vi "Test XY Scanning with Alazar.vi"() -> ()   [LabVIEW 2018]
uses:
  Hardware Mfg/AlazarTech SDK/Controls/Alazar Engine Actions.ctl
  <vilib>/ErrorRing/Error Ring.xnode
  General/Controls/Queue Manager Actions.ctl
  General/data manager action.ctl
  General/Controls/Optical Parameters.ctl
  General/Controls/Vibratome Parameters.ctl
  General/Controls/Translation Stage Types.ctl
  Hardware Mfg/Thorlabs Translation Stages/Controls/Translation Stage Cluster.ctl
  General/Controls/Translation Stage Parameters.ctl
  General/Controls/Scan Direction.ctl
  General/Controls/Imaging Parameters.ctl
  General/Controls/System Parameters.ctl
  Hardware Mfg/AlazarTech SDK/Controls/Clock Controls.ctl
  Hardware Mfg/AlazarTech SDK/Controls/Alazar Device ID.ctl
  Hardware Mfg/AlazarTech SDK/Controls/Channel Input Controls.ctl
  Hardware Mfg/AlazarTech SDK/Controls/Trigger Engine Controls.ctl
  Hardware Mfg/AlazarTech SDK/Controls/General Trigger Settings.ctl
  Hardware Mfg/AlazarTech SDK/Controls/Alazar Acquisition Settings.ctl
  General/type defines/file type.ctl
  General/Controls/Control cluster.ctl
panel:
  out "# save":i32
  out "# display":i32
  in  "save?":bool
  out "Image":T1(plugin-control)
  in  "Cluster":T2={"FFT value magnification"=1000.0, "max queue size (-1, unlimited)"=-1, "File Type"=enum."Tiff", "file path"=path "C:/Users/BoasLab/Documents/Data/Alazar data/B-line/data/test.tif", "#A-lines to save"=2048, "#Z pixels to save"=2048, "ImageDescription"="", "Convert to U16?"=FALSE} {"FFT value magnification" min=0.0 max=10000.0 step=0.001 format="%.4f"}
  out "error out":errorcluster
  in  "Acq Settings":T4={"Window Type"=1, "Record Length"=1440, "Footer"=0, "Output Format"=11, "Offset"=0, "Records Per Buffer"=2048, "Samples per record"=2048, "Records Count (Records/Acq)"=2147483647} {"Window Type" items=["DSP_WINDOW_NONE", "DSP_WINDOW_HANNING", "DSP_WINDOW_HAMMING", "DSP_WINDOW_BLACKMAN", "DSP_WINDOW_BLACKMAN_HARRIS", "DSP_WINDOW_BARTLETT"]; "Footer" items=["FOOTER_NONE", "FOOTER_NPT"]; "Output Format" items=["FLOAT_AMP2"=10, "FLOAT_LOG"=11]}
  in  "Trigger Settings":T7={"General Trigger Settings"={"Trigger Operation"=0, "Coupling ID"=2, "Range ID"=2, "Delay"=0, "Timeout Ticks"=0, "Mode"=1, "Parameter"=1}, "Trigger Engine 1"={"Trigger Engine"=0, "Source"=2, "Slope"=1, "Level"=140}, "Trigger Engine 2"={"Trigger Engine"=1, "Source"=3, "Slope"=1, "Level"=140}} {"General Trigger Settings"."Trigger Operation" items=["J", "K", "J OR K", "J AND K", "J XOR K", "J AND NOT K", "NOT J AND K"]; "General Trigger Settings"."Coupling ID" items=["AC"=1, "DC"=2]; "General Trigger Settings"."Range ID" items=["5 V", "1 V", "TTL"]; "Trigger Engine 1"."Trigger Engine" items=["J", "K"]; "Trigger Engine 1"."Source" items=["A", "B", "External", "Disable", "C", "D"]; "Trigger Engine 1"."Slope" items=["Positive"=1, "Negative"=2]; "Trigger Engine 2"."Trigger Engine" items=["J", "K"]; "Trigger Engine 2"."Source" items=["A", "B", "External", "Disable", "C", "D"]; "Trigger Engine 2"."Slope" items=["Positive"=1, "Negative"=2]}
  in  "Ch B Input Control":T8={"Channel"=2, "Coupling"=2, "Range"=10, "Impedance"=2} {"Channel" items=["A"=1, "B"=2, "C"=4, "D"=8]; "Coupling" items=["AC"=1, "DC"=2]; "Range" items=["20 mV"=1, "40 mV"=2, "50 mV"=3, "80 mV"=4, "100 mV"=5, "200 mV"=6, "400 mV"=7, "500 mV"=8, "800 mV"=9, "1 V"=10, "1.25 V"=33, "2 V"=11, "4 V"=12, "5 V"=13, "8 V"=14, "10 V"=15, "20 V"=16]; "Impedance" items=["1 MOhm"=1, "50 Ohm"=2, ""=0]}
  in  "Ch A Input Control":T8={"Channel"=1, "Coupling"=2, "Range"=10, "Impedance"=2} {"Channel" items=["A"=1, "B"=2, "C"=4, "D"=8]; "Coupling" items=["AC"=1, "DC"=2]; "Range" items=["20 mV"=1, "40 mV"=2, "50 mV"=3, "80 mV"=4, "100 mV"=5, "200 mV"=6, "400 mV"=7, "500 mV"=8, "800 mV"=9, "1 V"=10, "1.25 V"=33, "2 V"=11, "4 V"=12, "5 V"=13, "8 V"=14, "10 V"=15, "20 V"=16]; "Impedance" items=["1 MOhm"=1, "50 Ohm"=2, ""=0]}
  in  "Device ID":T9={"System ID"=1, "Board ID"=1}
  in  "Capture Clock":T10={"Sample Rate"=100, "Decimation"=0, "Source"=2, "Edge"=0} {"Edge" items=["Rising", "Falling"]; "Source" items=["Internal"=1, "Fast External"=2, "Medium External"=3, "Slow External"=4, "External AC"=5, "External DC"=6, "External 10MHz"=7]}
  out "Acquisition":i32
  in  "stop":bool
  in  "System Parameters":T11={"Optical Parameters"={"Obj. Focal Length [mm]"=45.0, "Scan Lens EFL[mm]"=59.5, "Tube Lens EFL[mm]"=205.0, "Galvo V Range (+/-)"=10.0, "Galvo Max Half Angle [Deg]"=19.0, "Max Galvo Range[%]"=0.0}, "Vibratome"={"Z Bottom [mm]"=0.0, "Pre Cut Dwell [s]"=0.0, "Blade Frequency [RPM]"=0, "Slice Speed [mm/s]"=0.0, "Post Cut Dwell [s]"=0.0, "Ramp Time [s]"=0.0, "Start X [mm]"=0.0, "Start Y [mm]"=0.0, "Slice Length [mm]"=0.0, "Slice Axis"=enum."Y Axis", "Controller VISA Ref"="COM4"}, "Table Stages"={"X Stage"={"Position"=0.0, "Is.Enabled?"=FALSE, "Is.Connected?"=FALSE, "Device SN"="45876539", "AccelerationMaximum"=0.0, "VelocityMaximum"=0.0, "Acceleration"=0.0, "Velocity"=0.0, "waitTimeout (ms)"=0, "Model"=enum."None", "Is.Homed?"=FALSE}, "Y Stage"={"Position"=0.0, "Is.Enabled?"=FALSE, "Is.Connected?"=FALSE, "Device SN"="45876539", "AccelerationMaximum"=0.0, "VelocityMaximum"=0.0, "Acceleration"=0.0, "Velocity"=0.0, "waitTimeout (ms)"=0, "Model"=enum."None", "Is.Homed?"=FALSE}, "Z Stage"={"Position"=0.0, "Is.Enabled?"=FALSE, "Is.Connected?"=FALSE, "Device SN"="45876539", "AccelerationMaximum"=0.0, "VelocityMaximum"=0.0, "Acceleration"=0.0, "Velocity"=0.0, "waitTimeout (ms)"=0, "Model"=enum."None", "Is.Homed?"=FALSE}}, "Imaging Parameter"={"Raster Scan Direction"=enum."Uni Directional", "Pixel Dwell Time [Clock Cycles]"=1, "Flyback Time [Clock Cycles]"=200, "XY Center [um]"={"X"=1.0, "Y"=1.0}, "Pixel Step Size [um]"=2.5, "XY Image Size"=enum."2048 x 2048", "Custom"=FALSE, "Custom Size"={"X"=10, "Y"=10}, "Line Averages"=1}} {"Imaging Parameter"."Line Averages" min=1 max=30 step=1; "Imaging Parameter"."Flyback Time [Clock Cycles]" max=1000 step=1; "Imaging Parameter"."Pixel Step Size [um]" min=0.0 max=10.0 step=0.01; "Imaging Parameter"."Custom Size"."Y" min=1 max=30 step=1; "Imaging Parameter"."Custom Size"."X" min=1 max=30 step=1; "Imaging Parameter"."XY Center [um]"."Y" min=1.0 max=30.0 step=1.0; "Imaging Parameter"."XY Center [um]"."X" min=1.0 max=30.0 step=1.0; "Imaging Parameter"."Pixel Dwell Time [Clock Cycles]" max=10 step=1}
  in  "Galvo HW Parameters":T19={"Analog Out Channel"="GalvoCtrl/ao0,GalvoCtrl/ao1", "Min Voltage"=-10.0, "Max Voltage"=10.0, "Pixel Clock Source"="/GalvoCtrl/PFI0", "Sample Rate"=1000.0, "Line Clock Out Ch"="GalvoCtrl/port0/line0"}
  # "X"
  # "X"
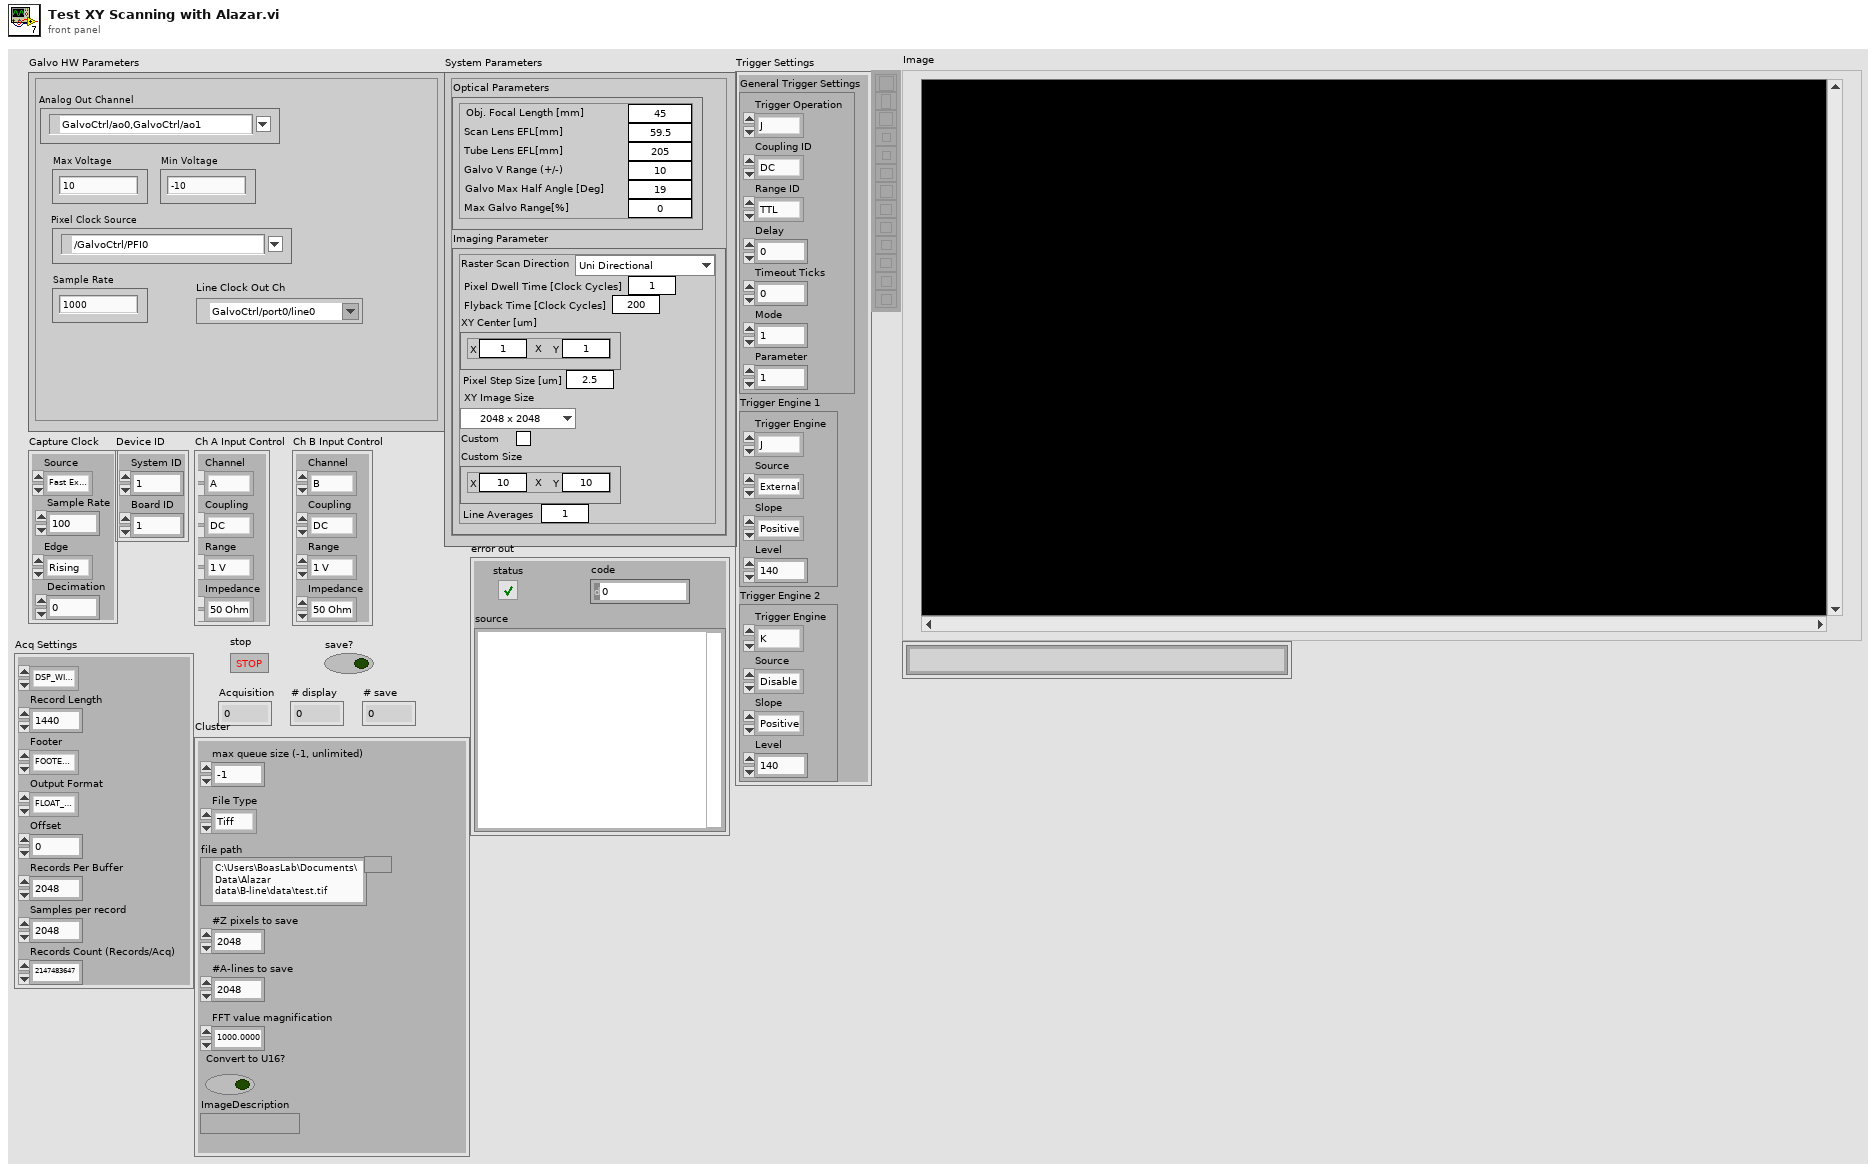
[diagram p1: front panel]
types:
  T1 = typedef "IMAQ Image.ctl" = refnum<image>
  T2 = typedef "Control cluster.ctl" = cluster{"FFT value magnification":dbl, "max queue size (-1, unlimited)":i32, "File Type":T3, "file path":path, "#A-lines to save":u32, "#Z pixels to save":u32, "ImageDescription":string, "Convert to U16?":bool}
  T3 = typedef "file type.ctl" = enum16{"text", "Tiff", "binary"}
  T4 = typedef "Alazar Acquisition Settings.ctl" = cluster{"Window Type":u32, "Record Length":u32, "Footer":u32, "Output Format":u32, "Offset":u32, "Records Per Buffer":u32, "Samples per record":u32, "Records Count (Records/Acq)":u32}
  T5 = typedef "General Trigger Settings.ctl" = cluster{"Trigger Operation":u32, "Coupling ID":u32, "Range ID":u32, "Delay":u32, "Timeout Ticks":u32, "Mode":u32, "Parameter":u32}
  T6 = typedef "Trigger Engine Controls.ctl" = cluster{"Trigger Engine":u32, "Source":u32, "Slope":u32, "Level":u32}
  T7 = cluster{"General Trigger Settings":T5, "Trigger Engine 1":T6, "Trigger Engine 2":T6}
  T8 = typedef "Channel Input Controls.ctl" = cluster{"Channel":u8, "Coupling":u32, "Range":u32, "Impedance":u32}
  T9 = typedef "Alazar Device ID.ctl" = cluster{"System ID":u32, "Board ID":u32}
  T10 = typedef "Clock Controls.ctl" = cluster{"Sample Rate":u32, "Decimation":u32, "Source":u32, "Edge":u32}
  T11 = typedef "System Parameters.ctl" = cluster{"Optical Parameters":T12, "Vibratome":T13, "Table Stages":T14, "Imaging Parameter":T17}
  T12 = typedef "Optical Parameters.ctl" = cluster{"Obj. Focal Length [mm]":dbl, "Scan Lens EFL[mm]":dbl, "Tube Lens EFL[mm]":dbl, "Galvo V Range (+/-)":dbl, "Galvo Max Half Angle [Deg]":dbl, "Max Galvo Range[%]":dbl}
  T13 = typedef "Vibratome Parameters.ctl" = cluster{"Z Bottom [mm]":dbl, "Pre Cut Dwell [s]":dbl, "Blade Frequency [RPM]":u16, "Slice Speed [mm/s]":dbl, "Post Cut Dwell [s]":dbl, "Ramp Time [s]":dbl, "Start X [mm]":dbl, "Start Y [mm]":dbl, "Slice Length [mm]":dbl, "Slice Axis":enum16{"X Axis", "Y Axis", "Z Axis"}, "Controller VISA Ref":refnum<visa-resource-name>}
  T14 = typedef "Translation Stage Parameters.ctl" = cluster{"X Stage":T15, "Y Stage":T15, "Z Stage":T15}
  T15 = typedef "Translation Stage Cluster.ctl" = cluster{"Position":dbl, "Is.Enabled?":bool, "Is.Connected?":bool, "Device SN":string, "AccelerationMaximum":dbl, "VelocityMaximum":dbl, "Acceleration":dbl, "Velocity":dbl, "waitTimeout (ms)":i32, "Model":T16, "Is.Homed?":bool}
  T16 = typedef "Translation Stage Types.ctl" = enum16{"None", "Thorlabs LTS", "Thorlabs MLJ"}
  T17 = typedef "Imaging Parameters.ctl" = cluster{"Raster Scan Direction":T18, "Pixel Dwell Time [Clock Cycles]":u16, "Flyback Time [Clock Cycles]":u16, "XY Center [um]":cluster{"X":dbl, "Y":dbl}, "Pixel Step Size [um]":dbl, "XY Image Size":enum16{"32 x 32", "64 x 64", "128 x 128", "256 x 256", "512 x 512", "1024 x 1024", "2048 x 2048"}, "Custom":bool, "Custom Size":cluster{"X":u16, "Y":u16}, "Line Averages":u8}
  T18 = typedef "Scan Direction.ctl" = enum16{"Uni Directional", "Bi Directional", "None"}
  T19 = cluster{"Analog Out Channel":tag, "Min Voltage":dbl, "Max Voltage":dbl, "Pixel Clock Source":tag, "Sample Rate":dbl, "Line Clock Out Ch":tag}
  T20 = typedef "Queue Manager Actions.ctl" = enum16{"Init", "Enqueue", "Enqueue All", "Preview Queue", "Dequeue", "Get Status", "Flush Queue", "Flush All Queues", "Release All Queues", "Release Queue", "Enqueue at Opposite End"}
  T21 = typedef "Alazar Engine Actions.ctl" = enum16{"Init", "Config Clock", "Config Ch", "Config Trig", "Config Non-FFT Acq.", "Non-FFT Acquire", "Load background from Non-FFT buffer", "enable background subtrac", "disable background subtrac", "load background from file", "load background from elsewhere", "start acquire", "background subtraction", "Config Acq.", "Acquire", "UnInit"}
  T22 = enum16{"Init", "Calc & Write Scan Pattern", "Start Galvo Task", "Is Task Done?", "Stop Galvo", "Uninit"}
  T23 = typedef "data manager action.ctl" = enum16{"Init: open file", "save", "save as text", "Uninit: close file"}
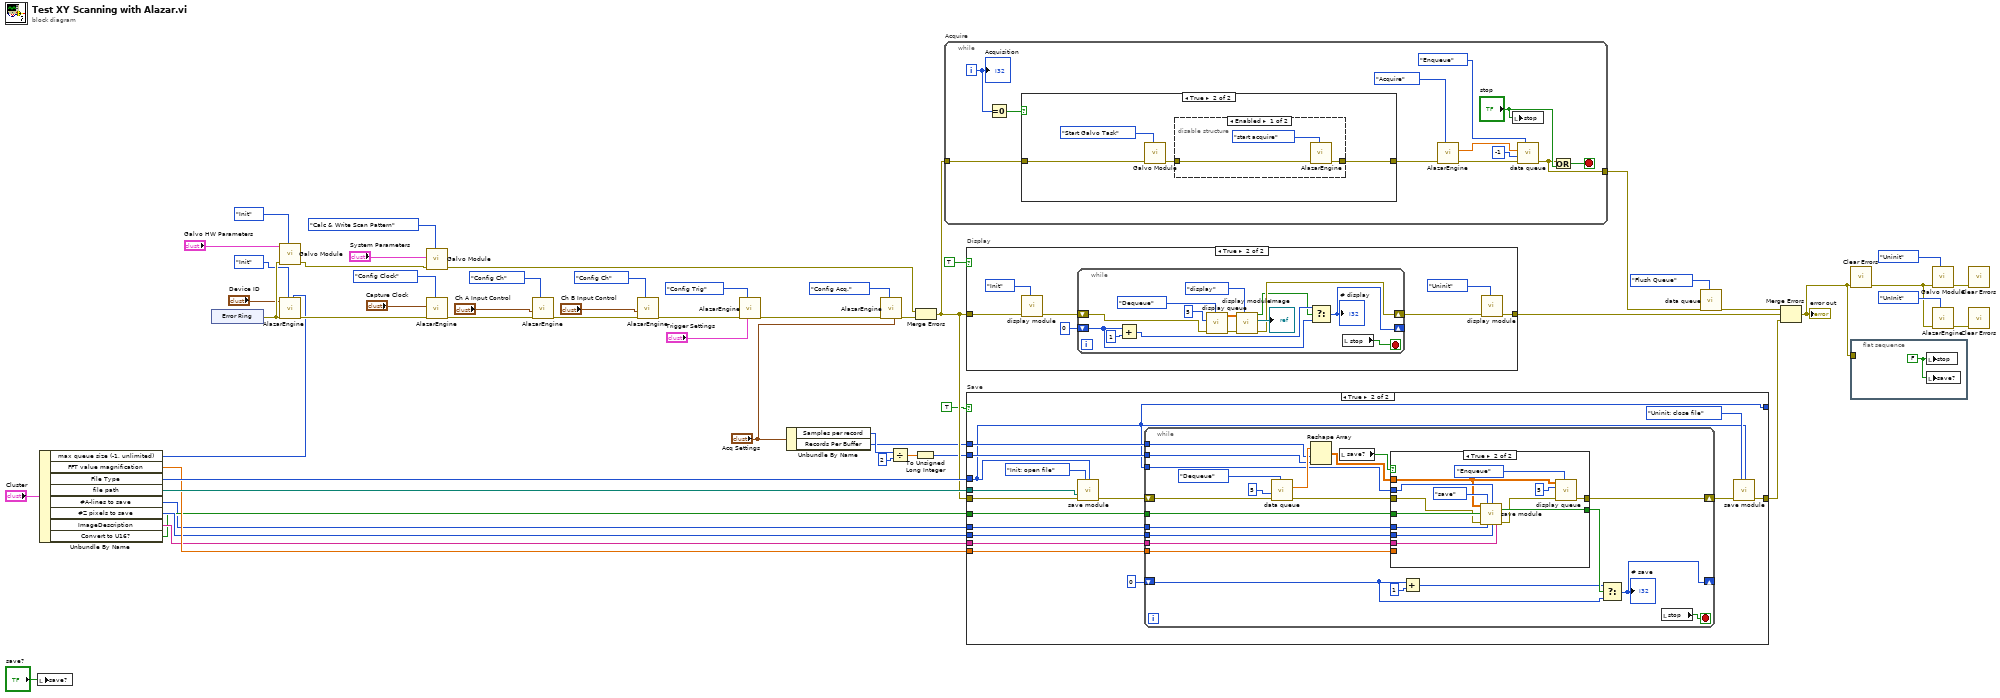
[diagram p0: block diagram]
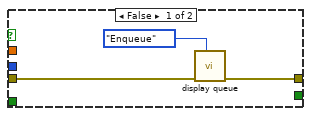
[diagram p3: hidden frame]
diagram:
  n1 = local write "save?"("save?") -> ()
  n2 = Unbundle By Name("Cluster") -> ("max queue size (-1, unlimited)"=w11:i32, "FFT value magnification"=w12:dbl, "File Type"=w16:T3, "file path"=w15:path, "#A-lines to save"=w3:u32, "#Z pixels to save"=w6:u32, "ImageDescription"=w5:string, "Convert to U16?"=w4:bool)
  n3 = xnode "Error Ring"() -> ("error out"=w45:errorcluster)
  n4 = call "Galvo Module.vi"("Action"=T22."Init", "error in (no error)"=w45, "Galvo HW Parameters"="Galvo HW Parameters") -> ("error out"=w52:errorcluster)  [unwired: 7 in, 1 out]
  n5 = call "AlazarEngine.vi"("max queue size (-1, unlimited)"=w11, "Action"=Alazar_Engine_Actions."Init", "error in (no error)"=w45, "Device ID"="Device ID") -> ("error out"=w48:errorcluster)  [unwired: 5 in, 2 out]
  n6 = call "Galvo Module.vi"("Action"=T22."Calc & Write Scan Pattern", "error in (no error)"=w52, "System Parameters"="System Parameters") -> ("error out"=w51:errorcluster)  [unwired: 7 in, 1 out]
  n7 = call "AlazarEngine.vi"("Action"=Alazar_Engine_Actions."Config Clock", "error in (no error)"=w48, "Capture Clock"="Capture Clock") -> ("error out"=w47:errorcluster)  [unwired: 6 in, 2 out]
  n8 = call "AlazarEngine.vi"("Action"=Alazar_Engine_Actions."Config Ch", "error in (no error)"=w47, "Ch Input Control"="Ch A Input Control") -> ("error out"=w46:errorcluster)  [unwired: 6 in, 2 out]
  n9 = call "AlazarEngine.vi"("Action"=Alazar_Engine_Actions."Config Ch", "error in (no error)"=w46, "Ch Input Control"="Ch B Input Control") -> ("error out"=w36:errorcluster)  [unwired: 6 in, 2 out]
  n10 = call "AlazarEngine.vi"("Trigger Settings"="Trigger Settings", "Action"=Alazar_Engine_Actions."Config Trig", "error in (no error)"=w36) -> ("error out"=w23:errorcluster)  [unwired: 6 in, 2 out]
  n11 = Unbundle By Name("Acq Settings") -> ("Samples per record"=w20:u32, "Records Per Buffer"=w1:u32)
  n12 = call "AlazarEngine.vi"("Acq Settings"="Acq Settings", "Action"=Alazar_Engine_Actions."Config Acq.", "error in (no error)"=w23) -> ("error out"=w32:errorcluster)  [unwired: 6 in, 2 out]
  n13 = Divide(x=w20, y=u32 2) -> (x/y=w18:dbl)
  n14 = To Unsigned Long Integer(number=w18) -> (unsigned 32bit integer=w2:u32)
  n15 = Merge Errors(w51, w32) -> (w10:errorcluster)
  n16 = while "Acquire" {
    tunnel: [w58] -> w24
    tunnel: w10 -> [w60]
    i -> [w59]
    stop <- w62 stop-if-true
    n17 = Equal To 0?(x=w59) -> (x = 0?=w66:bool)
    n18 = case shown="True" w66 {
      tunnel: [w67 w69] -> w65
      tunnel: w60 -> [w67 w68]
      frame False {
      }
      frame True {
        n19 = call "Galvo Module.vi"("Action"=T22."Start Galvo Task", "error in (no error)"=w68) -> ("error out"=w70:errorcluster)  [unwired: 8 in, 1 out]
        n20 = disable-structure shown="Enabled" {
          disable-tunnel: w70 -> [w74 w75]
          disable-tunnel: [w73 w75] -> w69
          frame Enabled {
            n21 = call "AlazarEngine.vi"("Action"=Alazar_Engine_Actions."start acquire", "error in (no error)"=w74) -> ("error out"=w73:errorcluster)  [unwired: 7 in, 2 out]
          }
          frame Disabled {
          }
        }
      }
    }
    n22 = call "AlazarEngine.vi"("Action"=Alazar_Engine_Actions."Acquire", "error in (no error)"=w65) -> ("error out"=w63:errorcluster, "Buffer"=w57:sgl[])  [unwired: 7 in, 1 out]
    n23 = local write "stop"("stop") -> ()
    n24 = call "data queue.vi"("Action"=Queue_Manager_Actions."Enqueue", "error in (no error)"=w63, "timeout in ms (-1)"=-1, "data in"=w57) -> ("error out"=w58:errorcluster)  [unwired: 4 in, 3 out]
    n25 = Or(x=w58, y="stop") -> (x .or. y?=w62:bool)
    "Acquisition" <- w59
  }
  n26 = case "Display" shown="True" TRUE {
    tunnel: [w76 w79] -> w14
    tunnel: w10 -> [w76 w78]
    frame False {
    }
    frame True {
      n27 = call "display module.vi"("Action"=enum16{"Init", "display", "Uninit"}."Init", "error in"=w78) -> ("error out"=w82:errorcluster)  [unwired: 7 in, 2 out]
      n28 = while {
        shift-right: [w94] -> w80
        shift-left: w82 -> [w88]
        shift-right: [w89] -> _
        shift-left: 0 -> [w90]
        stop <- w97 stop-if-true
        n29 = Add(x=w90, y=1) -> (x+y=w92:i32)
        n30 = call "display queue.vi"("Action"=Queue_Manager_Actions."Dequeue", "error in (no error)"=w88, "time out"=5 ("timeout in ms (-1)")) -> ("error out"=w85:errorcluster, "data out"=w84:sgl[][])  [unwired: 4 in, 3 out]
        n31 = call "display module.vi"("Action"=enum16{"Init", "display", "Uninit"}."display", "error in"=w85, "data in"=w84) -> ("error out"=w94:errorcluster, "Image"=→"Image":T1, "display successful?"=w91:bool)  [unwired: 6 in]
        n32 = Select(t=w92, s=w91, f=w90) -> (s? t:f=w89:i32)
        "# display" <- w89
        n33 = local read "stop"() -> (w97:bool)
      }
      n34 = call "display module.vi"("Action"=enum16{"Init", "display", "Uninit"}."Uninit", "error in"=w80) -> ("error out"=w79:errorcluster)  [unwired: 7 in, 2 out]
    }
  }
  n35 = case "Save" shown="True" TRUE {
    tunnel: w16 -> [_ w99]
    tunnel: w15 -> [_ w114]
    tunnel: [w98 w113] -> w13
    tunnel: w12 -> [_ w112]
    tunnel: w10 -> [w98 w111]
    tunnel: w6 -> [_ w107]
    tunnel: w5 -> [_ w104]
    tunnel: w4 -> [_ w105]
    tunnel: w3 -> [_ w106]
    tunnel: w2 -> [_ w103]
    tunnel: w1 -> [_ w102]
    tunnel: [_ w99] -> _
    frame False {
    }
    frame True {
      n36 = call "save module.vi"("action"=data_manager_action."Init: open file", "File Type"=w99, "file path and name"=w114, "error in (no error)"=w111) -> ("error out"=w110:errorcluster)  [unwired: 10 in, 1 out]
      n37 = while {
        tunnel: w112 -> [w135]
        shift-right: [w134] -> w109
        shift-left: w110 -> [w126]
        shift-right: [w129] -> _
        shift-left: 0 -> [w130]
        tunnel: w107 -> [w123]
        tunnel: w106 -> [w122]
        tunnel: w105 -> [w121]
        tunnel: w104 -> [w120]
        tunnel: w103 -> [w118]
        tunnel: w102 -> [w117]
        tunnel: w99 -> [w115]
        stop <- w136 stop-if-true
        n38 = call "data queue.vi"("Action"=Queue_Manager_Actions."Dequeue", "error in (no error)"=w126, "timeout in ms (-1)"=5) -> ("error out"=w124:errorcluster, "data out"=w119:sgl[])  [unwired: 5 in, 2 out]
        n39 = Reshape Array(w119, w117, w118) -> (w116:sgl[][])
        n40 = local read "save?"() -> (w125:bool)
        n41 = case shown="True" w125 {
          tunnel: w135 -> [_ _]
          tunnel: [w137 w140] -> w134
          tunnel: [_ w152] -> w133
          tunnel: w124 -> [w139 w142]
          tunnel: w123 -> [_ w149]
          tunnel: w122 -> [_ w148]
          tunnel: w121 -> [_ w147]
          tunnel: w120 -> [_ w146]
          tunnel: w116 -> [_ w143]
          tunnel: w115 -> [_ w144]
          frame False {
            n42 = call "display queue.vi"("Action"=Queue_Manager_Actions."Enqueue", "error in (no error)"=w139) -> ("error out"=w137:errorcluster)  [unwired: 5 in, 4 out]
          }
          frame True {
            n43 = call "save module.vi"("data in"=w143, "action"=data_manager_action."save", "File Type"=w144, "Convert to U16?"=w147, "error in (no error)"=w142, "# A-lines to save"=w148, "#Z pixels to save"=w149, "ImageDescription"=w146) -> ("save successful?"=w152:bool, "error out"=w141:errorcluster)  [unwired: 6 in]
            n44 = call "display queue.vi"("Action"=Queue_Manager_Actions."Enqueue", "error in (no error)"=w141, "time out"=5, "data in"=w143) -> ("error out"=w140:errorcluster)  [unwired: 3 in, 4 out]
          }
        }
        n45 = Add(x=w130, y=1) -> (x+y=w131:i32)
        n46 = Select(t=w131, s=w133, f=w130) -> (s? t:f=w129:i32)
        "# save" <- w129
        n47 = local read "stop"() -> (w136:bool)
      }
      n48 = call "save module.vi"("action"=data_manager_action."Uninit: close file", "File Type"=w99, "error in (no error)"=w109) -> ("error out"=w113:errorcluster)  [unwired: 11 in, 1 out]
    }
  }
  n49 = call "data queue.vi"("Action"=Queue_Manager_Actions."Flush Queue", "error in (no error)"=w24) -> ("error out"=w22:errorcluster)  [unwired: 6 in, 3 out]
  n50 = Merge Errors(w22, w14, w13) -> (w26:errorcluster)
  "error out" <- w26
  n51 = call <vilib>:"Clear Errors.vi"("error in (no error)"=w26) -> ("error out"=w29:errorcluster)  [unwired: 5 in, 1 out]
  n52 = flat-sequence {
    tunnel: w26 -> [_]
    frame #0 {
      w153 = FALSE ("stop")
      n53 = local write "stop"(w153) -> ()
      n54 = local write "save?"(w153) -> ()
    }
  }
  n55 = call "Galvo Module.vi"("Action"=T22."Uninit", "error in (no error)"=w29) -> ("error out"=w28:errorcluster)  [unwired: 8 in, 1 out]
  n56 = call "AlazarEngine.vi"("Action"=Alazar_Engine_Actions."UnInit", "error in (no error)"=w29) -> ("error out"=w27:errorcluster)  [unwired: 7 in, 2 out]
  n57 = call <vilib>:"Clear Errors.vi"("error in (no error)"=w28) -> ()  [unwired: 5 in, 2 out]
  n58 = call <vilib>:"Clear Errors.vi"("error in (no error)"=w27) -> ()  [unwired: 5 in, 2 out]
